vi "Draw.vi"(8 "error in (no error)":errorcluster, 9 "Highlighted":string, 10 "picture in":picture, 11 "FSM in":refnum<class "FSM.Node.lvclass">) -> (0 "error out":errorcluster, 2 "picture out":picture, 3 "FSM out":refnum<class "FSM.Node.lvclass">)   [LabVIEW 2015, in "FSM.Node.lvclass"]
uses:
  FSM.Node.lvclass
  FSM.Node.lvclass/FSM.Node.ctl
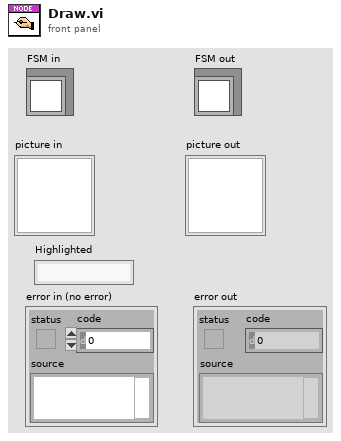
[diagram p1: front panel]
types:
  T1 = cluster{"Font Name:":string, "Size":i16, "Strikeout?":bool, "Italic?":bool, "Underline?":bool, "Outline?":bool, "Shadow?":bool, "Bold?":bool}
  T2 = cluster{"horizontal":enum16{"left", "center", "right"}, "vertical":enum16{"top", "center", "bottom"}}
  T3 = cluster{"Width":i16, "Style":enum32{"Solid", "Dash", "Dot", "DashDot", "DashDotDot"}}
  T4 = typedef "FSM.Node.lvclass/Shape.ctl" = enum16{"Default", "Start", "Action", "End"}
  T5 = cluster{"left":i16, "top":i16, "right":i16, "bottom":i16}
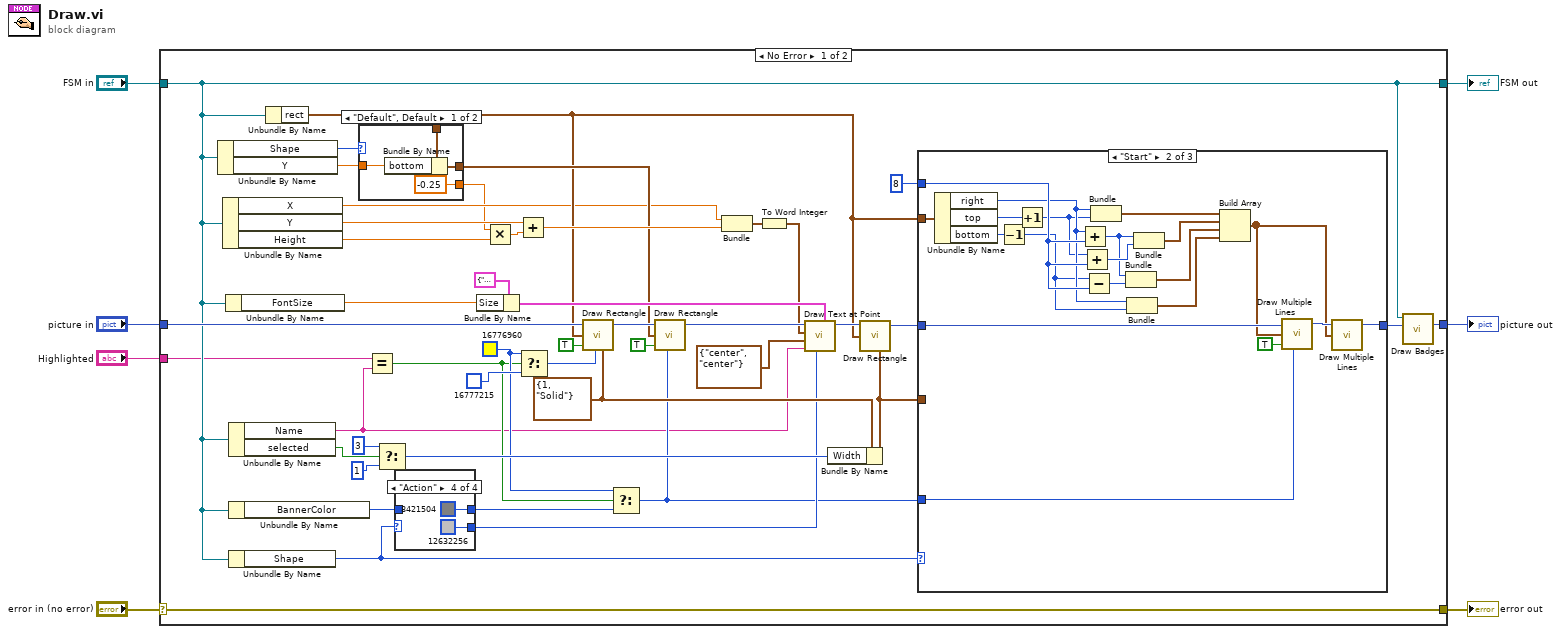
[diagram p0: block diagram]
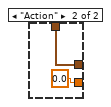
[diagram p2: hidden frame]
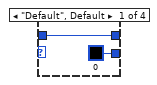
[diagram p3: hidden frame]
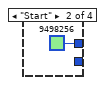
[diagram p4: hidden frame]
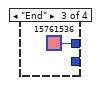
[diagram p5: hidden frame]
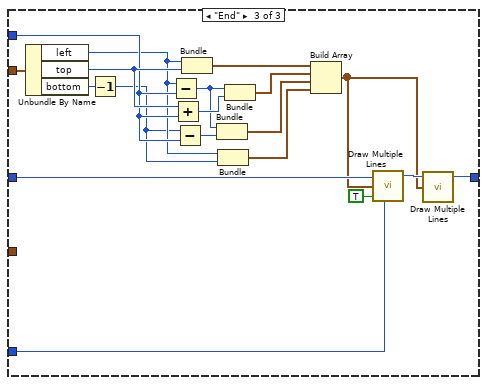
[diagram p7: hidden frame]
diagram:
  n1 = case shown="No Error" "error in (no error)" {
    selector: "error in (no error)" -> [w52 w107]
    tunnel: [w52 w107] -> w6
    tunnel: [w16 w106] -> w4
    tunnel: "FSM in" -> [w16 w106]
    tunnel: "picture in" -> [w51 w105]
    tunnel: [w17 w105] -> w2
    tunnel: "Highlighted" -> [w13 _]
    frame No Error {
      w10 = u32 16776960 ("color(black)")
      w48 = T3 {"Width"=1, "Style"=enum."Solid"} ("pen")
      n2 = Unbundle By Name(w16) -> ("Shape"=w26:T4, "Y"=w36:dbl)
      n3 = Unbundle By Name(w16) -> ("X"=w24:dbl, "Y"=w23:dbl, "Height"=w22:dbl)
      n4 = Unbundle By Name(w16) -> ("FontSize"=w42:dbl)
      n5 = Unbundle By Name(w16) -> ("Name"=w8:string, "selected"=w35:bool)
      n6 = Unbundle By Name(w16) -> ("BannerColor"=w29:u32)
      n7 = Unbundle By Name(w16) -> ("Shape"=w28:T4)
      n8 = Unbundle By Name(w16) -> ("rect"=w25:T5)
      n9 = case shown="\"Default\", Default" w26 {
        tunnel: [w56 w58] -> w37
        tunnel: w36 -> [w55 _]
        tunnel: w25 -> [w54 w58]
        tunnel: [-0.25 0.0] -> w19
        frame "Default", Default {
          n10 = Bundle By Name(cluster=w54, "bottom"=w55) -> (w56:T5)
        }
        frame "Action" {
        }
      }
      n11 = Equal?(x=w13, y=w8) -> (x = y?=w9:bool)
      n12 = Select(t=i16 3 ("Width"), s=w35, f=i16 1 ("Width")) -> (s? t:f=w32:i16)
      n13 = case shown="\"Action\"" w28 {
        tunnel: w29 -> [w60 _ _ _]
        tunnel: [w60 u32 9498256 u32 15761536 u32 8421504] -> w12
        tunnel: [u32 0 _ _ u32 12632256] -> w21
        frame "Default", Default {
        }
        frame "Start" {
        }
        frame "End" {
        }
        frame "Action" {
        }
      }
      n14 = Bundle By Name(cluster=T1 {"Font Name:"="Arial", "Size"=12, "Strikeout?"=FALSE, "Italic?"=FALSE, "Underline?"=FALSE, "Outline?"=FALSE, "Shadow?"=FALSE, "Bold?"=FALSE} ("[user-specified font]"), "Size"=w42) -> (w43:T1)
      n15 = Multiply(x=w19, y=w22) -> (x*y=w20:dbl)
      n16 = Add(x=w23, y=w20) -> (x+y=w39:dbl)
      n17 = Select(t=w10, s=w9, f=u32 16777215 ("color(black)")) -> (s? t:f=w14:u32)
      n18 = call <vilib>:"Draw Rectangle.vi"("picture"=w51, "rect"=w25, "fill?(F)"=TRUE, "color(black)"=w14, "pen"=w48) -> ("new picture"=w49:picture)  [unwired: 4 in]
      n19 = Select(t=w10, s=w9, f=w12) -> (s? t:f=w11:u32)
      n20 = call <vilib>:"Draw Rectangle.vi"("picture"=w49, "rect"=w37, "fill?(F)"=TRUE, "color(black)"=w11) -> ("new picture"=w46:picture)  [unwired: 5 in]
      n21 = Bundle("X"=w24, w39) -> (w40:cluster{"X":dbl, dbl})  [unwired: 1 in]
      n22 = To Word Integer(number=w40) -> (16bit integer=w38:cluster{"X":i16, i16})
      n23 = call <vilib>:"Draw Text at Point.vi"("[user-specified font]"=w43, "text color(black)"=w21, "text"=w8, "alignment(left, top)"=T2 {"horizontal"=enum."center", "vertical"=enum."center"}, "origin"=w38, "picture"=w46) -> ("new picture"=w41:picture)  [unwired: 4 in, 1 out]
      n24 = Bundle By Name(cluster=w48, "Width"=w32) -> (w27:T3)
      n25 = call <vilib>:"Draw Rectangle.vi"("picture"=w41, "rect"=w25, "pen"=w27) -> ("new picture"=w31:picture)  [unwired: 6 in]
      n26 = case shown="\"Start\"" w28 {
        tunnel: w31 -> [w65 w74 w93]
        tunnel: [w65 w69 w88] -> w18
        tunnel: w25 -> [_ w85 w104]
        tunnel: 8 -> [_ w82 w101]
        tunnel: w11 -> [_ w72 w91]
        tunnel: w27 -> [_ _ _]
        frame "Default", Default {
        }
        frame "Start" {
          n27 = Unbundle By Name(w85) -> ("right"=w79:i16, "top"=w84:i16, "bottom"=w78:i16)
          n28 = Decrement(x=w78) -> (x-1=w66:i16)
          n29 = Increment(x=w84) -> (x+1=w67:i16)
          n30 = Add(x=w79, y=w82) -> (x+y=w80:i32)
          n31 = Add(x=w67, y=w82) -> (x+y=w83:i32)
          n32 = Subtract(x=w66, y=w82) -> (x-y=w81:i32)
          n33 = Bundle("right"=w79, w67) -> (w68:cluster{"right":i16, i16})  [unwired: 1 in]
          n34 = Bundle(w80, w81) -> (w76:cluster{i32, i32})  [unwired: 1 in]
          n35 = Bundle("right"=w79, w66) -> (w75:cluster{"right":i16, i16})  [unwired: 1 in]
          n36 = Bundle(w80, w83) -> (w77:cluster{i32, i32})  [unwired: 1 in]
          n37 = Build Array(w68, w77, w76, w75) -> (w70:cluster{"right":i32, i32}[])
          n38 = call <vilib>:"Draw Multiple Lines.vi"("picture"=w74, "line endpoints"=w70, "fill?(F)"=TRUE, "color(black)"=w72) -> ("new picture"=w71:picture)  [unwired: 5 in]
          n39 = call <vilib>:"Draw Multiple Lines.vi"("picture"=w71, "line endpoints"=w70) -> ("new picture"=w69:picture)  [unwired: 7 in]
        }
        frame "End" {
          n40 = Unbundle By Name(w104) -> ("left"=w98:i16, "top"=w103:i16, "bottom"=w97:i16)
          n41 = Decrement(x=w97) -> (x-1=w86:i16)
          n42 = Subtract(x=w98, y=w101) -> (x-y=w99:i32)
          n43 = Add(x=w103, y=w101) -> (x+y=w102:i32)
          n44 = Subtract(x=w86, y=w101) -> (x-y=w100:i32)
          n45 = Bundle("left"=w98, "top"=w103) -> (w87:cluster{"left":i16, "top":i16})  [unwired: 1 in]
          n46 = Bundle(w99, w100) -> (w95:cluster{i32, i32})  [unwired: 1 in]
          n47 = Bundle("left"=w98, w86) -> (w94:cluster{"left":i16, i16})  [unwired: 1 in]
          n48 = Bundle(w99, w102) -> (w96:cluster{i32, i32})  [unwired: 1 in]
          n49 = Build Array(w87, w96, w95, w94) -> (w89:cluster{"left":i32, "top":i32}[])
          n50 = call <vilib>:"Draw Multiple Lines.vi"("picture"=w93, "line endpoints"=w89, "fill?(F)"=TRUE, "color(black)"=w91) -> ("new picture"=w90:picture)  [unwired: 5 in]
          n51 = call <vilib>:"Draw Multiple Lines.vi"("picture"=w90, "line endpoints"=w89) -> ("new picture"=w88:picture)  [unwired: 7 in]
        }
      }
      n52 = call "Draw Badges.vi"("picture in"=w18, "FSM in"=w16) -> ("picture out"=w17:picture)  [unwired: 7 in, 2 out]
    }
    frame Error {
    }
  }
  "error out" <- w6
  "FSM out" <- w4
  "picture out" <- w2
